vi "WT210 Element Data.vi"(0 "VISA Refnum in":refnum<visa-resource-name>, 2 "Dryer PowerData in":T1 {"Voltage (V):Element 1 Avg" format="%.3g"; "Voltage (V):Element 2 Avg" format="%.3g"; "Max Watt Hours" format="%.3g"; "Power Factor:Element 2" format="%.3g"; "Power Factor:Element 1" format="%.3g"; "Apparent Power (VA):Element 2" format="%.3g"; "Apparent Power (VA):Element 1" format="%.3g"; "Frequency (Hz):Element 1" format="%.3g"; "Time:Element 1" format="%.3g"; "Voltage Crest Factor:Element 2" format="%.3g"; "Voltage Crest Factor:Element 1" format="%.3g"; "Voltage Harmonic (%):Element 2" format="%.3g"; "Voltage Harmonic (%):Element 1" format="%.3g"; "Current Crest Factor:Element 2" format="%.3g"; "Current Crest Factor:Element 1" format="%.3g"; "Voltage (V):Element 1" format="%.3g"; "Voltage (V):Element 2" format="%.3g"; "Watt Hours (Wh):Sigma" format="%.3f"; "Power (W):Sigma" format="%.3g"; "Current (A):Element 2" format="%.3e"; "Current (A):Element 1" format="%.3e"}, 3 "C Factor (0: V)":u16, 5 "error in (no error)":errorcluster, 6 "V Range (6: 600V)":u16(ring)=4 items=["Auto", "15V", "30V", "60V", "150V", "300V", "600V"], 8 "Element (1: Element 1)":u16, 9 "Uthd:Element 1":dbl, 10 "C Factor (0: V) 2":u16, 11 "Uthd:Element 2":dbl, 12 "A Range (12: 20A)":u16(ring)=10 items=["Auto", "5mA", "10mA", "20mA", "50mA", "100mA", "200mA", "0.5A", "1A", "2A", "5A", "10A", "20A", "50mV", "100mV", "200mV", "2.5V", "5V", "10V"]) -> (14 "VISA Refnum out":refnum<visa-resource-name>, 16 "Dryer PowerData out":T1 {"Voltage (V):Element 1 Avg" format="%.3g"; "Voltage (V):Element 2 Avg" format="%.3g"; "Max Watt Hours" format="%.3g"; "Power Factor:Element 2" format="%.3g"; "Power Factor:Element 1" format="%.3g"; "Apparent Power (VA):Element 2" format="%.3g"; "Apparent Power (VA):Element 1" format="%.3g"; "Frequency (Hz):Element 1" format="%.3g"; "Time:Element 1" format="%.3g"; "Voltage Crest Factor:Element 2" format="%.3g"; "Voltage Crest Factor:Element 1" format="%.3g"; "Voltage Harmonic (%):Element 2" format="%.3g"; "Voltage Harmonic (%):Element 1" format="%.3g"; "Current Crest Factor:Element 2" format="%.3g"; "Current Crest Factor:Element 1" format="%.3g"; "Voltage (V):Element 1" format="%.3g"; "Voltage (V):Element 2" format="%.3g"; "Watt Hours (Wh):Sigma" format="%.3f"; "Power (W):Sigma" format="%.3g"; "Current (A):Element 2" format="%.3e"; "Current (A):Element 1" format="%.3e"}, 19 "error out":errorcluster)   [LabVIEW 2020]
uses:
  Trunk/Utility/Type Definitions/UTILITY Power Data.ctl
  Yokogawa WT200 Series.lvlib
panel:
  out "Error Counter":u32
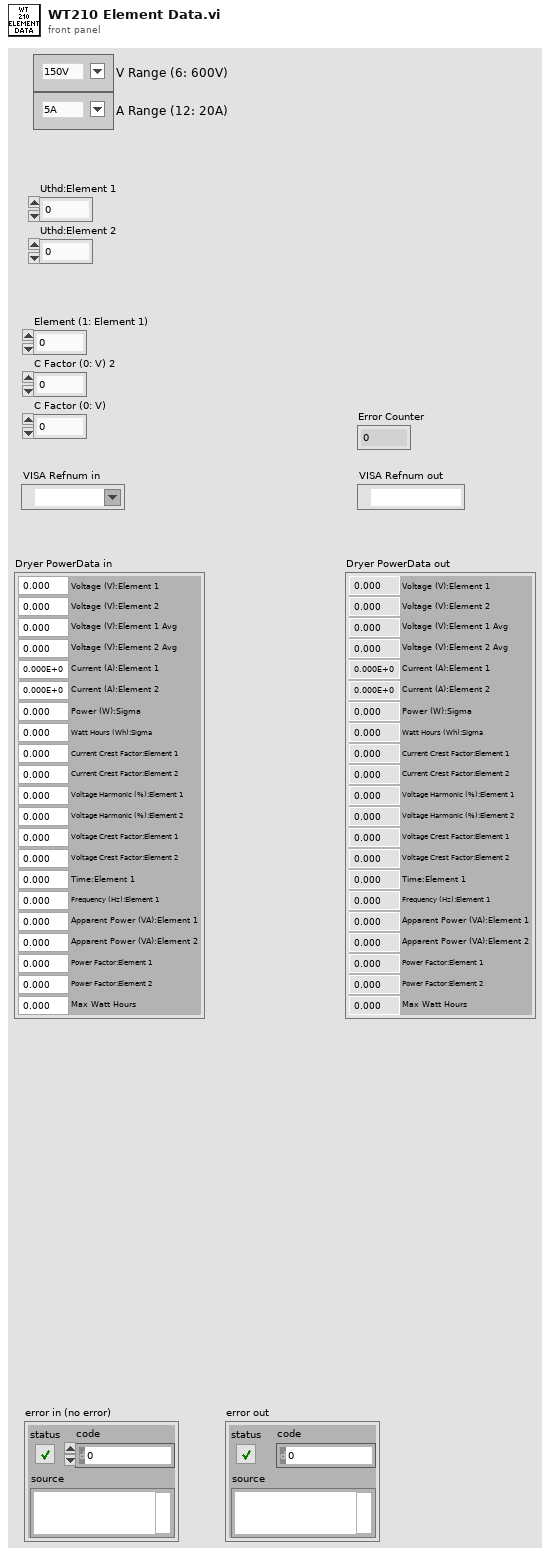
[diagram p1: front panel]
types:
  T1 = typedef "UTILITY Power Data.ctl" = cluster{"Current (A):Element 1":dbl, "Current (A):Element 2":dbl, "Power (W):Sigma":dbl, "Watt Hours (Wh):Sigma":dbl, "Voltage (V):Element 2":dbl, "Voltage (V):Element 1":dbl, "Current Crest Factor:Element 1":dbl, "Current Crest Factor:Element 2":dbl, "Voltage Harmonic (%):Element 1":dbl, "Voltage Harmonic (%):Element 2":dbl, "Voltage Crest Factor:Element 1":dbl, "Voltage Crest Factor:Element 2":dbl, "Time:Element 1":dbl, "Frequency (Hz):Element 1":dbl, "Apparent Power (VA):Element 1":dbl, "Apparent Power (VA):Element 2":dbl, "Power Factor:Element 1":dbl, "Power Factor:Element 2":dbl, "Max Watt Hours":dbl, "Voltage (V):Element 2 Avg":dbl, "Voltage (V):Element 1 Avg":dbl}
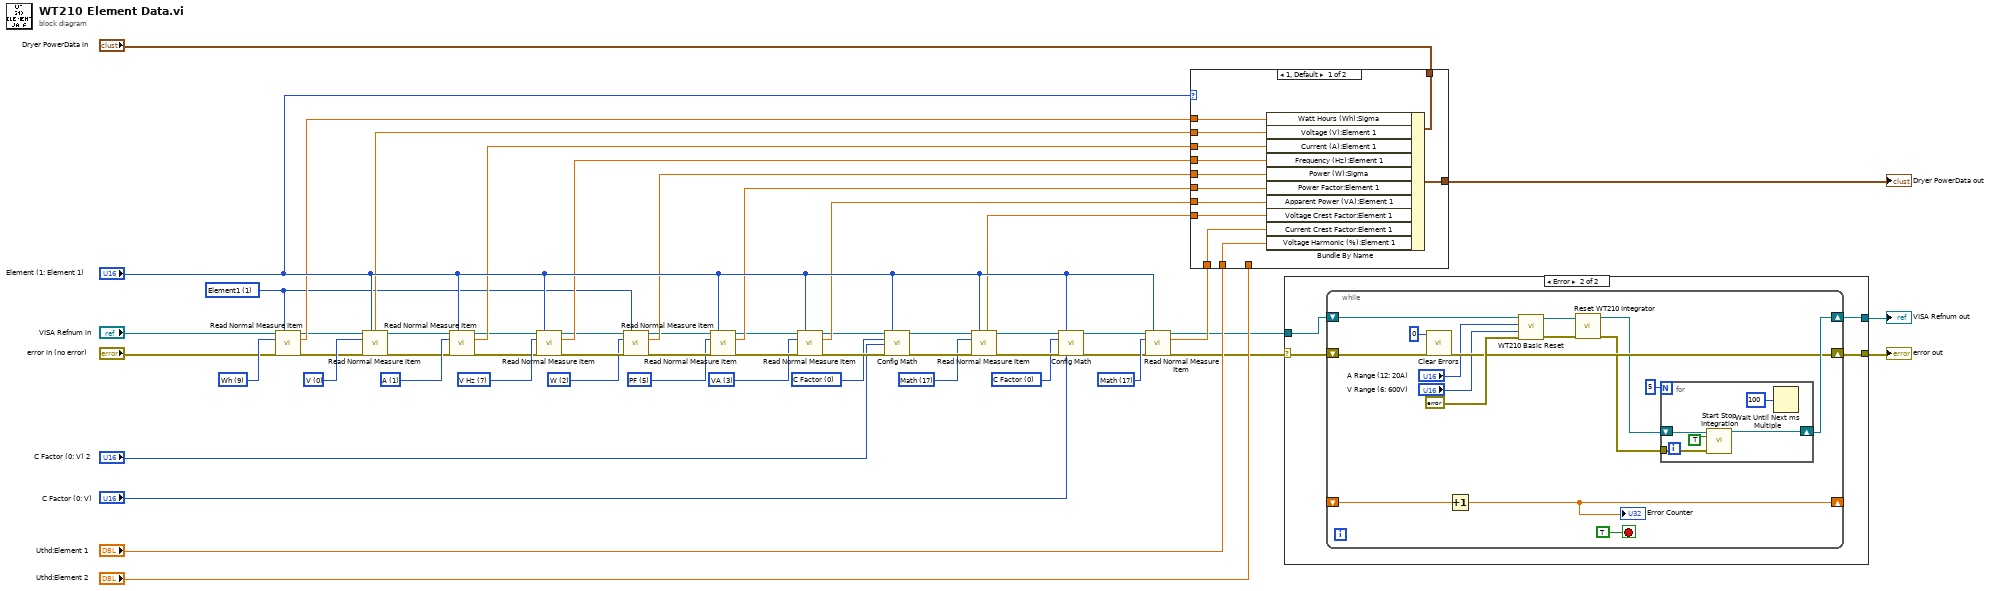
[diagram p0: block diagram]
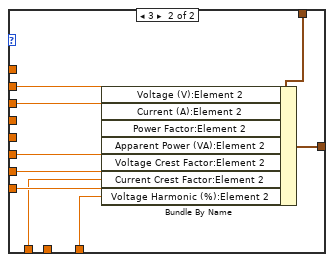
[diagram p3: hidden frame]
diagram:
  w5 = u16 1 items=["", "Element1", "Element2", "Element3", "Sigma"] ("Element (1: Element 1)")
  w41 = u16 17 items=["V", "A", "W", "VA", "var", "PF", "deg", "V Hz", "A Hz", "Wh", "Wh+", "Wh-", "Ah", "Ah+", "Ah-", "Vpk", "Apk", "Math"] ("Measure Item (0: V)")
  w36 = u16 0 items=["C Factor", "Arithmetic", "Average", "Efficiency"] ("Math Type (0: Crest Factor)")
  w31 = u16 0 items=["C Factor", "Arithmetic", "Average", "Efficiency"] ("Math Type (0: Crest Factor)")
  w29 = u16 17 items=["V", "A", "W", "VA", "var", "PF", "deg", "V Hz", "A Hz", "Wh", "Wh+", "Wh-", "Ah", "Ah+", "Ah-", "Vpk", "Apk", "Math"] ("Measure Item (0: V)")
  w22 = u16 3 items=["V", "A", "W", "VA", "var", "PF", "deg", "V Hz", "A Hz", "Wh", "Wh+", "Wh-", "Ah", "Ah+", "Ah-", "Vpk", "Apk", "Math"] ("Measure Item (0: V)")
  w21 = u16 5 items=["V", "A", "W", "VA", "var", "PF", "deg", "V Hz", "A Hz", "Wh", "Wh+", "Wh-", "Ah", "Ah+", "Ah-", "Vpk", "Apk", "Math"] ("Measure Item (0: V)")
  w20 = u16 2 items=["V", "A", "W", "VA", "var", "PF", "deg", "V Hz", "A Hz", "Wh", "Wh+", "Wh-", "Ah", "Ah+", "Ah-", "Vpk", "Apk", "Math"] ("Measure Item (0: V)")
  w19 = u16 7 items=["V", "A", "W", "VA", "var", "PF", "deg", "V Hz", "A Hz", "Wh", "Wh+", "Wh-", "Ah", "Ah+", "Ah-", "Vpk", "Apk", "Math"] ("Measure Item (0: V)")
  w18 = u16 1 items=["V", "A", "W", "VA", "var", "PF", "deg", "V Hz", "A Hz", "Wh", "Wh+", "Wh-", "Ah", "Ah+", "Ah-", "Vpk", "Apk", "Math"] ("Measure Item (0: V)")
  w17 = u16 0 items=["V", "A", "W", "VA", "var", "PF", "deg", "V Hz", "A Hz", "Wh", "Wh+", "Wh-", "Ah", "Ah+", "Ah-", "Vpk", "Apk", "Math"] ("Measure Item (0: V)")
  w10 = u16 9 items=["V", "A", "W", "VA", "var", "PF", "deg", "V Hz", "A Hz", "Wh", "Wh+", "Wh-", "Ah", "Ah+", "Ah-", "Vpk", "Apk", "Math"] ("Measure Item (0: V)")
  n1 = call "Read Normal Measure Item.vi"("VISA resource name"="VISA Refnum in", "Element (1: Element 1)"=w5, "Measure Item (0: V)"=w10, "error in (no error)"="error in (no error)") -> ("VISA resource name out"=w16:refnum<visa-resource-name>, "Measure Value"=w52:sgl, "error out"=w13:errorcluster)  [unwired: 9 in]
  n2 = call "Read Normal Measure Item.vi"("VISA resource name"=w16, "Element (1: Element 1)"="Element (1: Element 1)", "Measure Item (0: V)"=w17, "error in (no error)"=w13) -> ("VISA resource name out"=w14:refnum<visa-resource-name>, "Measure Value"=w44:sgl, "error out"=w11:errorcluster)  [unwired: 9 in]
  n3 = call "Read Normal Measure Item.vi"("VISA resource name"=w14, "Element (1: Element 1)"="Element (1: Element 1)", "Measure Item (0: V)"=w18, "error in (no error)"=w11) -> ("VISA resource name out"=w15:refnum<visa-resource-name>, "Measure Value"=w43:sgl, "error out"=w12:errorcluster)  [unwired: 9 in]
  n4 = call "Read Normal Measure Item.vi"("VISA resource name"=w15, "Element (1: Element 1)"="Element (1: Element 1)", "Measure Item (0: V)"=w19, "error in (no error)"=w12) -> ("VISA resource name out"=w28:refnum<visa-resource-name>, "Measure Value"=w46:sgl, "error out"=w25:errorcluster)  [unwired: 9 in]
  n5 = call "Read Normal Measure Item.vi"("VISA resource name"=w28, "Element (1: Element 1)"=w5, "Measure Item (0: V)"=w20, "error in (no error)"=w25) -> ("VISA resource name out"=w26:refnum<visa-resource-name>, "Measure Value"=w47:sgl, "error out"=w23:errorcluster)  [unwired: 9 in]
  n6 = call "Read Normal Measure Item.vi"("VISA resource name"=w26, "Element (1: Element 1)"="Element (1: Element 1)", "Measure Item (0: V)"=w21, "error in (no error)"=w23) -> ("VISA resource name out"=w27:refnum<visa-resource-name>, "Measure Value"=w48:sgl, "error out"=w24:errorcluster)  [unwired: 9 in]
  n7 = call "Read Normal Measure Item.vi"("VISA resource name"=w27, "Element (1: Element 1)"="Element (1: Element 1)", "Measure Item (0: V)"=w22, "error in (no error)"=w24) -> ("VISA resource name out"=w34:refnum<visa-resource-name>, "Measure Value"=w49:sgl, "error out"=w32:errorcluster)  [unwired: 9 in]
  n8 = call "Config Math.vi"("VISA resource name"=w34, "Element (1: Element 1)"="Element (1: Element 1)", "Math Type (0: Crest Factor)"=w31, "C Factor (0: V)"="C Factor (0: V) 2", "error in (no error)"=w32) -> ("VISA resource name out"=w35:refnum<visa-resource-name>, "error out"=w33:errorcluster)  [unwired: 9 in]
  n9 = call "Read Normal Measure Item.vi"("VISA resource name"=w35, "Element (1: Element 1)"="Element (1: Element 1)", "Measure Item (0: V)"=w29, "error in (no error)"=w33) -> ("VISA resource name out"=w42:refnum<visa-resource-name>, "Measure Value"=w50:sgl, "error out"=w38:errorcluster)  [unwired: 9 in]
  n10 = call "Config Math.vi"("VISA resource name"=w42, "Element (1: Element 1)"="Element (1: Element 1)", "Math Type (0: Crest Factor)"=w36, "C Factor (0: V)"="C Factor (0: V)", "error in (no error)"=w38) -> ("VISA resource name out"=w39:refnum<visa-resource-name>, "error out"=w40:errorcluster)  [unwired: 9 in]
  n11 = call "Read Normal Measure Item.vi"("VISA resource name"=w39, "Element (1: Element 1)"="Element (1: Element 1)", "Measure Item (0: V)"=w41, "error in (no error)"=w40) -> ("VISA resource name out"=w4:refnum<visa-resource-name>, "Measure Value"=w45:sgl, "error out"=w2:errorcluster)  [unwired: 9 in]
  n12 = case shown="1, Default" "Element (1: Element 1)" {
    tunnel: [w66 w74] -> w8
    tunnel: "Dryer PowerData in" -> [w65 w75]
    tunnel: w43 -> [w64 w72]
    tunnel: w44 -> [w63 w73]
    tunnel: w45 -> [w62 w68]
    tunnel: w46 -> [w61 _]
    tunnel: w47 -> [w60 _]
    tunnel: w48 -> [w59 w71]
    tunnel: w49 -> [w58 w70]
    tunnel: w50 -> [w57 w69]
    tunnel: "Uthd:Element 1" -> [w56 _]
    tunnel: w52 -> [w55 _]
    tunnel: "Uthd:Element 2" -> [_ w67]
    frame 1, Default {
      n13 = Bundle By Name(cluster=w65, "Watt Hours (Wh):Sigma"=w55, "Voltage (V):Element 1"=w63, "Current (A):Element 1"=w64, "Frequency (Hz):Element 1"=w61, "Power (W):Sigma"=w60, "Power Factor:Element 1"=w59, "Apparent Power (VA):Element 1"=w58, "Voltage Crest Factor:Element 1"=w57, "Current Crest Factor:Element 1"=w62, "Voltage Harmonic (%):Element 1"=w56) -> (w66:T1)
    }
    frame 3 {
      n14 = Bundle By Name(cluster=w75, "Voltage (V):Element 2"=w73, "Current (A):Element 2"=w72, "Power Factor:Element 2"=w71, "Apparent Power (VA):Element 2"=w70, "Voltage Crest Factor:Element 2"=w69, "Current Crest Factor:Element 2"=w68, "Voltage Harmonic (%):Element 2"=w67) -> (w74:T1)
    }
  }
  "Dryer PowerData out" <- w8
  n15 = case shown="Error" w2 {
    selector: w2 -> [w77 w80]
    tunnel: w4 -> [w76 w81]
    tunnel: [w76 w79] -> w3
    tunnel: [w77 w78] -> w1
    frame No Error {
    }
    frame Error {
      n16 = while {
        shift-right: [w93] -> w79
        shift-left: w81 -> [w97]
        shift-right: [w92] -> w78
        shift-left: w80 -> [w95]
        shift-right: [w87] -> _
        shift-left: _ -> [w88]
        stop <- TRUE stop-if-true
        n17 = call <vilib>:"Clear Errors.vi"("error in (no error)"=w95, "specific error code to clear (0: all)"=0) -> ("error out"=w92:errorcluster)  [unwired: 4 in, 1 out]
        n18 = Increment(x=w88) -> (x+1=w87:dbl)
        "Error Counter" <- w87
        n19 = call "WT210 Basic Reset.vi"("error in (no error)"=errorcluster {"status"=FALSE, "code"=0, "source"=""}, "V Range (6: 600V)"="V Range (6: 600V)", "A Range (12: 20A)"="A Range (12: 20A)", "VISA Refnum in"=w97) -> ("error out"=w85:errorcluster, "VISA Refnum out"=w86:refnum<visa-resource-name>)  [unwired: 4 in, 2 out]
        n20 = call "Reset WT210 Integrator.vi"("error in (no error)"=w85, "VISA resource name"=w86) -> ("error out"=w84:errorcluster, "VISA resource name out"=w83:refnum<visa-resource-name>)  [unwired: 8 in]
        n21 = for {
          N: 5 -> [_]
          tunnel: w84 -> [w100]
          shift-right: [w101] -> w93
          shift-left: w83 -> [w99]
          n22 = call "Start Stop Integration.vi"("VISA resource name"=w99, "Start/Stop (F: Stop)"=TRUE, "error in (no error)"=w100) -> ("VISA resource name out"=w101:refnum<visa-resource-name>)  [unwired: 11 in, 1 out]
          n23 = Wait Until Next ms Multiple(millisecond multiple=u32 100) -> ()  [unwired: 1 out]
        }
      }
    }
  }
  "error out" <- w1
  "VISA Refnum out" <- w3
